vi "best_angle.vi"(3 "Waypoint Heading":dbl, 4 "Current Heading":dbl, 5 "Wind Vector":cluster{"Wind Speed":dbl, "Wind Theta":dbl}) -> (0 "Heading Candidate 2":dbl, 1 "Heading Candidate 1":dbl, 2 "Best Angle":dbl)   [LabVIEW 2011]
doc: "Takes the absolute wind vector, the heading of your next waypoint, and your current heading, and recommends a heading.\n\nWe repeatedly run the iterate theta VI until its outputs converge. The converging outputs are the two angles which minimize the travel time to the waypoint.\n\nAfter the while loop, we determine which angle is closer to the current heading. We choose the closer heading unless the other heading has a significantly higher dr/dt."
panel:
  in  "thres+":dbl=2.0
  in  "thresh x":dbl=1.2
  # "Inputs"
  # "Outputs"
  # "Constants to determine when to tack"
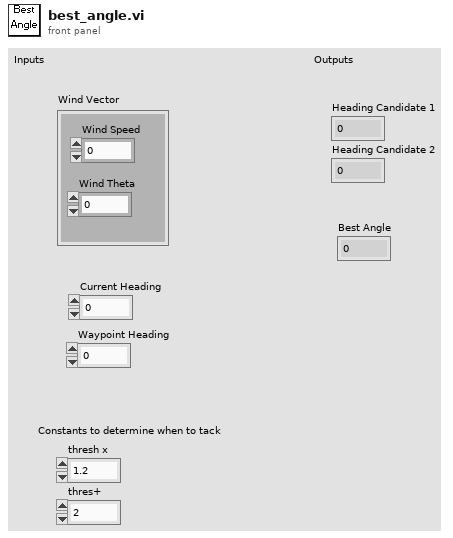
[diagram p1: front panel]
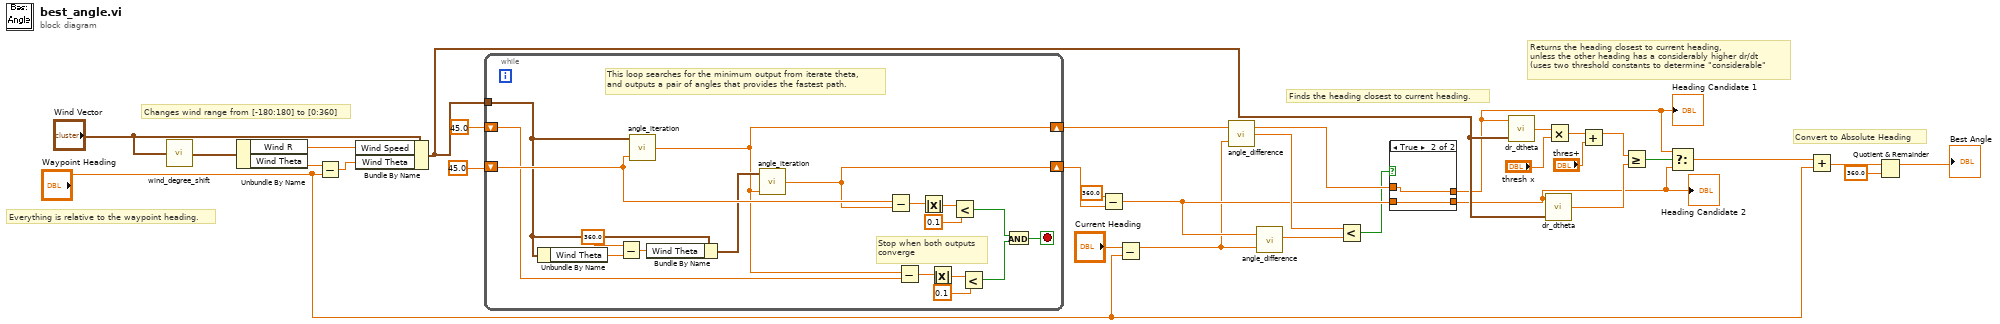
[diagram p0: block diagram]
diagram:
  # "Returns the heading closest to current heading,\nunless the other heading has a considerably higher dr/dt\n(uses two threshold constants to determine \"considerable\""
  # "Finds the heading closest to current heading."
  # "Changes wind range from [-180:180] to [0:360]"
  # "Convert to Absolute Heading"
  # "Everything is relative to the waypoint heading."
  n1 = call "wind_degree_shift.vi"("Wind Vector -180 - 180"="Wind Vector") -> ("Wind Vector 0-360"=w23:cluster{"Wind R":dbl, "Wind Theta":dbl})
  n2 = Unbundle By Name(w23) -> ("Wind R"=w22:dbl, "Wind Theta"=w20:dbl)
  n3 = Subtract(x=w20, y="Waypoint Heading") -> (x-y=w21:dbl)
  n4 = Bundle By Name(cluster="Wind Vector", "Wind Speed"=w22, "Wind Theta"=w21) -> (w8:cluster{"Wind Speed":dbl, "Wind Theta":dbl})
  n5 = while {
    shift-right: [w45] -> w27
    shift-left: 45.0 ("Best Theta") -> [w46]
    tunnel: w8 -> [w34]
    shift-right: [w32] -> w14
    shift-left: 45.0 ("Best Theta") -> [w41]
    stop <- w38 stop-if-true
    # "This loop searches for the minimum output from iterate theta,\nand outputs a pair of angles that provides the fastest path."
    # "Stop when both outputs\nconverge"
    n6 = Unbundle By Name(w34) -> ("Wind Theta"=w36:dbl)
    n7 = Subtract(x=360.0, y=w36) -> (x-y=w33:dbl)
    n8 = call "angle_iteration.vi"("Phi"=w46, "Wind Vector"=w34) -> ("Best Theta"=w32:dbl)  [unwired: 1 in]
    n9 = Bundle By Name(cluster=w34, "Wind Theta"=w33) -> (w35:cluster{"Wind Speed":dbl, "Wind Theta":dbl})
    n10 = call "angle_iteration.vi"("Phi"=w32, "Wind Vector"=w35) -> ("Best Theta"=w45:dbl)  [unwired: 1 in]
    n11 = Subtract(x=w46, y=w45) -> (x-y=w49:dbl)
    n12 = Subtract(x=w32, y=w41) -> (x-y=w42:dbl)
    n13 = Absolute Value(x=w49) -> (abs(x)=w48:dbl)
    n14 = Absolute Value(x=w42) -> (abs(x)=w43:dbl)
    n15 = Less?(x=w48, y=0.1) -> (x < y?=w40:bool)
    n16 = Less?(x=w43, y=0.1) -> (x < y?=w39:bool)
    n17 = And(x=w40, y=w39) -> (x .and. y?=w38:bool)
  }
  n18 = Subtract(x=360.0, y=w27) -> (x-y=w13:dbl)
  n19 = Subtract(x="Current Heading", y="Waypoint Heading") -> (x-y=w7:dbl)
  n20 = call "angle_difference.vi"("Angle 2"=w7, "Angle 1"=w14) -> ("Difference"=w25:dbl)
  n21 = call "angle_difference.vi"("Angle 2"=w7, "Angle 1"=w13) -> ("Difference"=w26:dbl)
  n22 = Less?(x=w25, y=w26) -> (x < y?=w12:bool)
  n23 = case shown="True" w12 {
    tunnel: w14 -> [w51 w53]
    tunnel: [w50 w53] -> w2
    tunnel: [w51 w52] -> w1
    tunnel: w13 -> [w50 w52]
    frame False {
    }
    frame True {
    }
  }
  "Heading Candidate 1" <- w2
  "Heading Candidate 2" <- w1
  n24 = call "dr_dtheta.vi"("Wind Vector"=w8, "Boat Angle"=w2) -> ("dr/dt"=w19:dbl)  [unwired: 1 in]
  n25 = call "dr_dtheta.vi"("Wind Vector"=w8, "Boat Angle"=w1) -> ("dr/dt"=w16:dbl)  [unwired: 1 in]
  n26 = Multiply(x=w19, y="thresh x") -> (x*y=w15:dbl)
  n27 = Add(x=w15, y="thres+") -> (x+y=w11:dbl)
  n28 = Greater Or Equal?(x=w11, y=w16) -> (x >= y?=w17:bool)
  n29 = Select(t=w2, s=w17, f=w1) -> (s? t:f=w30:dbl)
  n30 = Add(x=w30, y="Waypoint Heading") -> (x+y=w5:dbl)
  n31 = Quotient & Remainder(x=w5, y=360.0) -> (x-y*floor(x/y)=→"Best Angle":dbl)  [unwired: 1 out]
